vi "Do.vi"(8 "error in (no error)":errorcluster, 10 "Actor in":refnum<class "Actor.lvclass">, 11 "EMS Set Device Parameter Status Msg":refnum<class "EMS Set Device Parameter Status Msg.lvclass">) -> (0 "error out":errorcluster, 2 "Actor out":refnum<class "Actor.lvclass">)   [LabVIEW 2015, in "Master Controller Core.lvlib" / "EMS Set Device Parameter Status Msg.lvclass"]
doc: "This VI delivers the message to the actor by calling the appropriate method(s) on the actor."
uses:
  EMS Set Device Parameter Status Msg.lvclass
  <vilib>/ActorFramework/Actor/Actor.lvclass
  Master Controller/Master Controller.lvclass
  SCADA Core/SCADA Abstract Messages/Set Device Parameter Status Msg/Set Device Parameter Status Msg.lvclass/Set Device Parameter Status Msg.ctl
  SCADA Core/SCADA Abstract Messages/Set Device Parameter Status Msg/Set Device Parameter Status Msg.lvclass
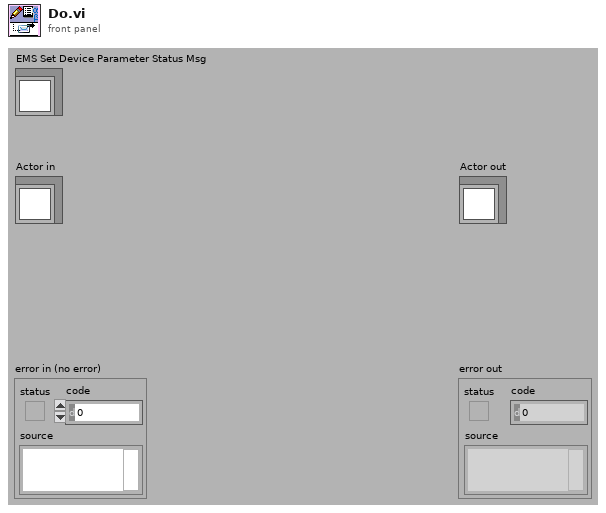
[diagram p1: front panel]
types:
  T1 = typedef "SCADA Core.lvlib/Set Device Parameter Status Msg.lvclass/Set Device Parameter Status.ctl" = enum16{"Success", "Failure"}
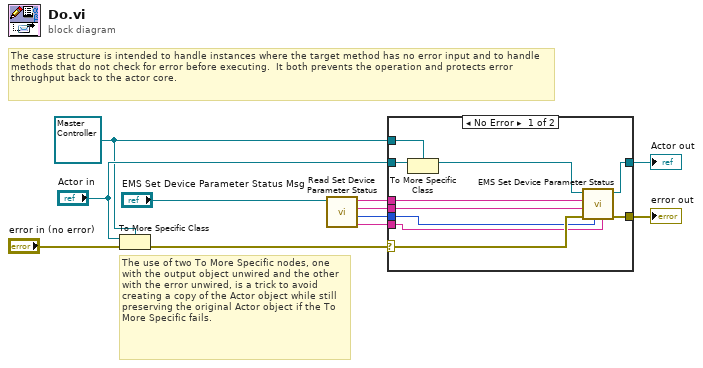
[diagram p0: block diagram]
diagram:
  w6 = refnum<class "Master Controller.lvclass"> refnum ("Actor in")
  # "The use of two To More Specific nodes, one with the output object unwired and the other with the error unwired, is a trick to avoid creating a copy of the Actor object while still preserving the original Actor object if the To More Specific fails."
  # "The case structure is intended to handle instances where the target method has no error input and to handle methods that do not check for error before executing.  It both prevents the operation and protects error throughput back to the actor core."
  n1 = To More Specific Class(target class=w6, reference="Actor in", error in="error in (no error)") -> (error out=w10:errorcluster)  [unwired: 1 out]
  n2 = call "Read Set Device Parameter Status.vi"("Set Device Parameter Status Msg in"="EMS Set Device Parameter Status Msg") -> ("error"=w1:string, "Status"=w2:T1, "Parameter Name"=w3:string, "IED Name"=w4:string)  [unwired: 6 in, 1 out]
  n3 = case shown="No Error" w10 {
    selector: w10 -> [w19 w23]
    tunnel: [w21 w23] -> w9
    tunnel: [w20 w22] -> w8
    tunnel: "Actor in" -> [w18 w22]
    tunnel: w6 -> [w17 _]
    tunnel: w4 -> [w15 _]
    tunnel: w3 -> [w14 _]
    tunnel: w2 -> [w13 _]
    tunnel: w1 -> [w12 _]
    frame No Error {
      n4 = To More Specific Class(target class=w17, reference=w18) -> (specific class reference=w16:refnum<class "Master Controller.lvclass">)  [unwired: 1 in, 1 out]
      n5 = call-dynamic "EMS Set Device Parameter Status.vi"("error"=w12, "Status"=w13, "error in (no error)"=w19, "Parameter Name"=w14, "IED Name"=w15, "Master Controller in"=w16) -> ("error out"=w21:errorcluster, "Master Controller out"=w20:refnum<class "Master Controller.lvclass">)  [unwired: 4 in]
    }
    frame Error {
      # "If type check fails, pass the original object out again."
    }
  }
  "error out" <- w9
  "Actor out" <- w8
